vi "FT10_Connect Fornax Handler.vi"(8 "error in (no error)":errorcluster, 10 "Message Data":variant, 11 "Message Handling Cluster in":T1) -> (0 "error out":errorcluster, 2 "Fornax Connected?":bool, 3 "Message Handling Cluster out":T1)   [LabVIEW 2024]
doc: "Opens or closes TCP connection to Fornax."
uses:
  Controls/Control_Message Handling Cluster.ctl
  Controls/Control_M4X Connection.ctl
  Controls/Control_PXI-7854R FPGA Reference.ctl
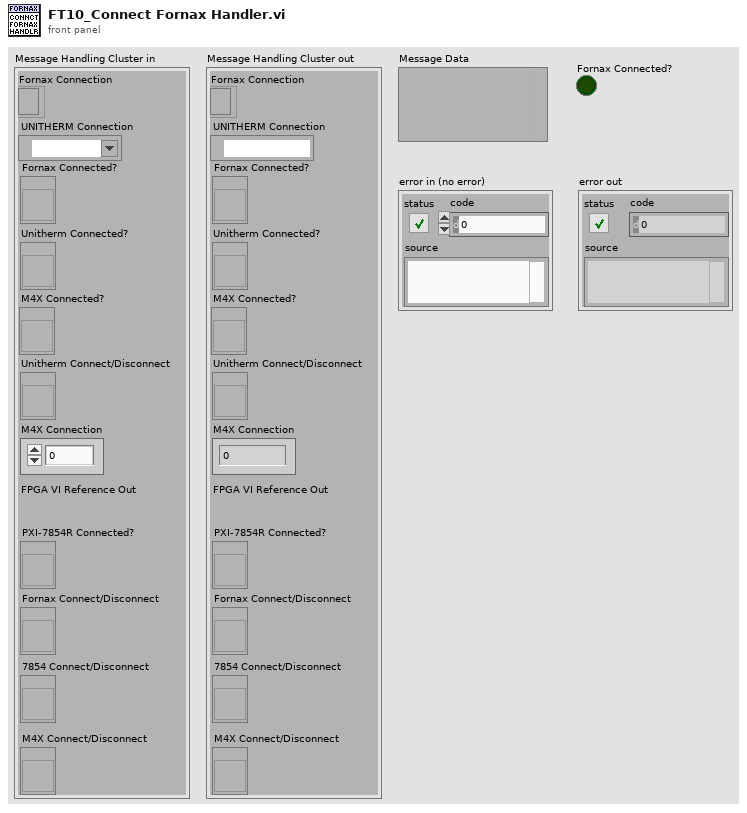
[diagram p1: front panel]
types:
  T1 = typedef "Control_Message Handling Cluster.ctl" = cluster{"Fornax Connected?":refnum<vi>, "Unitherm Connected?":refnum<vi>, "M4X Connected?":refnum<vi>, "Unitherm Connect/Disconnect":refnum<vi>, "Fornax Connection":refnum<k5>, "UNITHERM Connection":refnum<visa-resource-name>, "M4X Connection":T2, "PXI-7854R FPGA Reference":T3, "PXI-7854R Connected?":refnum<vi>, "Fornax Connect/Disconnect":refnum<vi>, "7854 Connect/Disconnect":refnum<vi>, "M4X Connect/Disconnect":refnum<vi>}
  T2 = typedef "Control_M4X Connection.ctl" = u32
  T3 = typedef "Control_PXI-7854R FPGA Reference.ctl" = refnum<k20>
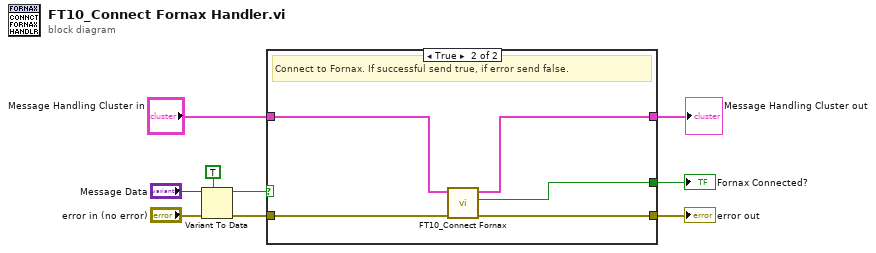
[diagram p0: block diagram]
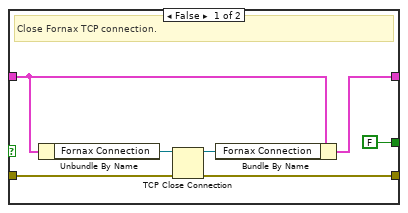
[diagram p2: hidden frame]
diagram:
  n1 = Variant To Data(error in="error in (no error)", type=TRUE, Variant="Message Data") -> (data=w2:bool, error out=w3:errorcluster)
  n2 = case shown="True" w2 {
    tunnel: [w11 w20] -> w9
    tunnel: [w15 w17] -> w6
    tunnel: "Message Handling Cluster in" -> [w16 w18]
    tunnel: w3 -> [w12 w21]
    tunnel: [FALSE w19] -> w1
    frame False {
      # "Close Fornax TCP connection."
      n3 = Unbundle By Name(w16) -> ("Fornax Connection"=w14:refnum<k5>)
      n4 = TCP Close Connection(connection ID=w14, error in (no error)=w12) -> (connection ID out=w13:refnum<k5>, error out=w11:errorcluster)  [unwired: 1 in]
      n5 = Bundle By Name(cluster=w16, "Fornax Connection"=w13) -> (w15:T1)
    }
    frame True {
      # "Connect to Fornax. If successful send true, if error send false."
      n6 = call "FT10_Connect Fornax.vi"("error in (no error)"=w21, "Message Handling Cluster in"=w18) -> ("error out"=w20:errorcluster, "Fornax Connected?"=w19:bool, "Message Handling Cluster out"=w17:T1)  [unwired: 7 in]
    }
  }
  "error out" <- w9
  "Message Handling Cluster out" <- w6
  "Fornax Connected?" <- w1
